vi "Write Sweep Speed (Hz).vi"(8 "error in (no error)":errorcluster, 10 "Sweep Speed (Hz)":dbl, 11 "Laser in":refnum<class "Laser.lvclass">) -> (0 "error out":errorcluster, 3 "Laser out":refnum<class "Laser.lvclass">)   [LabVIEW 2015, in "Laser.lvclass"]
uses:
  Laser.lvclass
  Laser.lvclass/Laser.ctl
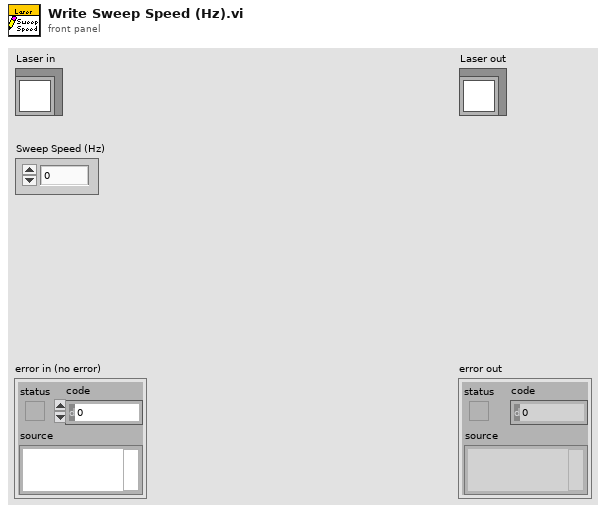
[diagram p1: front panel]
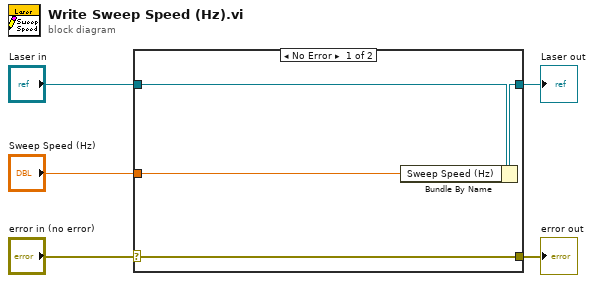
[diagram p0: block diagram]
diagram:
  n1 = case shown="No Error" "error in (no error)" {
    selector: "error in (no error)" -> [w9 w10]
    tunnel: [w9 w10] -> w4
    tunnel: [w7 w11] -> w2
    tunnel: "Laser in" -> [w8 w11]
    tunnel: "Sweep Speed (Hz)" -> [w6 _]
    frame No Error {
      n2 = Bundle By Name(cluster=w8, "Sweep Speed (Hz)"=w6) -> (w7:refnum<class "Laser.lvclass">)
    }
    frame Error {
    }
  }
  "error out" <- w4
  "Laser out" <- w2
